vi "FestoCPX.DO.Data.Fglb.vi"(6 "Config":T1[](array[typedef]), 7 "state (get all)":T4=enum."get", 8 "error in (no error)":errorcluster, 9 "State":bool[](array[boolean]), 10 "Outputs":T3[](array[typedef])) -> (0 "error out":errorcluster, 1 "changed?":bool, 2 "State out":bool[](array[boolean]))   [LabVIEW 2016]
uses:
  FestoCPX.DO.Data.Fglb.Action.ctl
  FestoCPX.DO.Signal.ctl
  FestoCPX.DO.Sets.ctl
  FestoCPX.DO.ctl
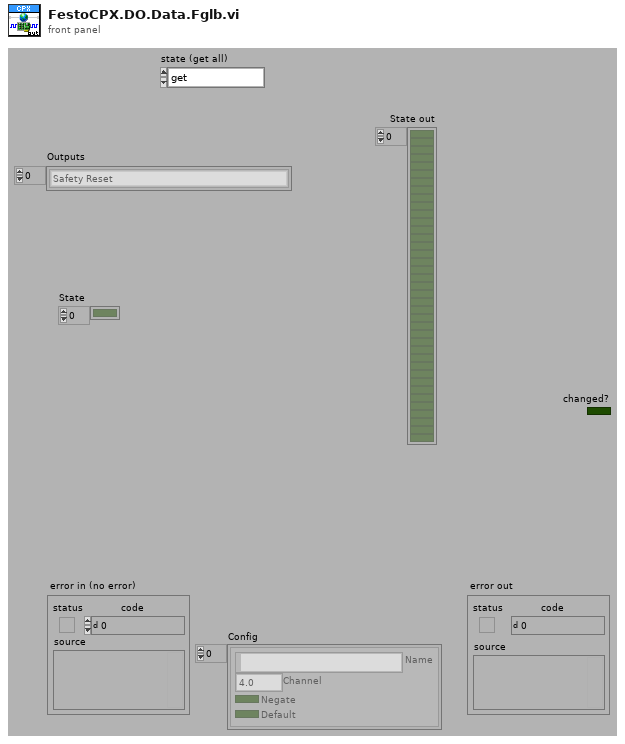
[diagram p1: front panel]
types:
  T1 = typedef "FestoCPX.DO.Sets.ctl" = cluster{"Name":string, "Channel":T2, "Negate":bool, "Default":bool}
  T2 = typedef "FestoCPX.DO.ctl" = enum16{"4.0", "4.1", "4.2", "4.3", "4.4", "4.5", "4.6", "4.7", "5.0", "5.1", "5.2", "5.3", "5.4", "5.5", "5.6", "5.7", "6.0", "6.1", "6.2", "6.3", "6.4", "6.5", "6.6", "6.7", "Q1K1", "Q1K2", "Q2K1", "Q2K2", "Q3K1", "Q3K2", "Q4K1", "Q4K2", "Q5K1", "Q5K2", "Q6K1", "Q6K2"}
  T3 = typedef "FestoCPX.DO.Signal.ctl" = enum16{"Safety Reset", "Air Main Valve", "Door Lock", "Button LED Start", "Button LED Stop", "Button LED Control", "Traffic LED Red", "Traffic LED Orange", "Traffic LED Green", "Horn", "Laser Interlock", "Laser Trigger", "Laser Fume Extractor", "Product Suction Gripper Slot 1 A", "Product Suction Gripper Slot 1 B", "Product Suction Gripper Slot 2 A", "Product Suction Gripper Slot 2 B", "Product Suction Gripper Slot 3 A", "Product Suction Gripper Slot 3 B", "Product Suction Gripper Slot 4 A", "Product Suction Gripper Slot 4 B", "Product Suction Gripper Final A", "Product Suction Gripper Final B", "Lamp", "Q1 Product Move Work", "Q1 Product Move Home", "Q2 Table Turn Work", "Q2 Table Turn Home", "Q3 Product Lift A", "Q3 Product Lift B", "Q4 Product Arm OK", "Q4 Product Arm NOK", "Q5 Product Arm Work", "Q6 Product BlowOut A", "Q6 Product BlowOut B"}
  T4 = typedef "FestoCPX.DO.Data.Fglb.Action.ctl" = enum16{"init", "set", "get", "check", "select", "reset"}
  T5 = cluster{"out":bool[], "Config":T1[], "changed":bool}
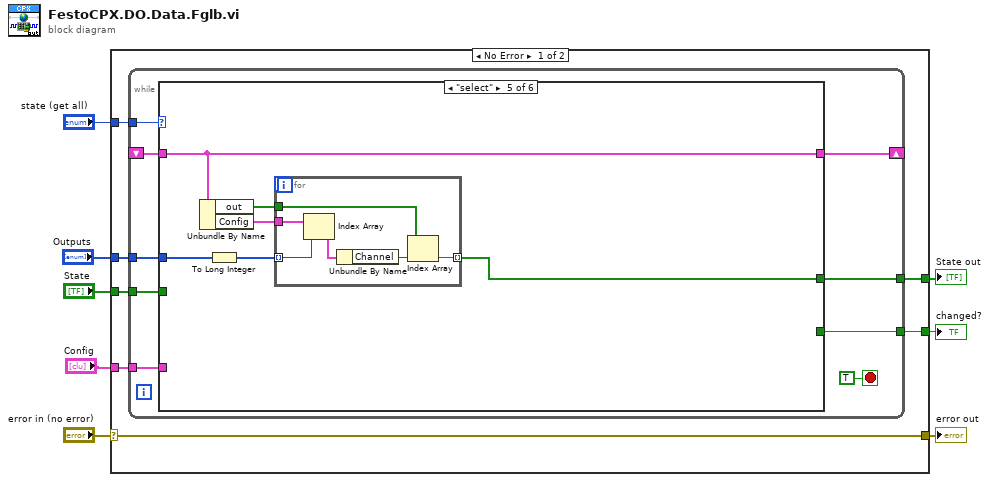
[diagram p0: block diagram]
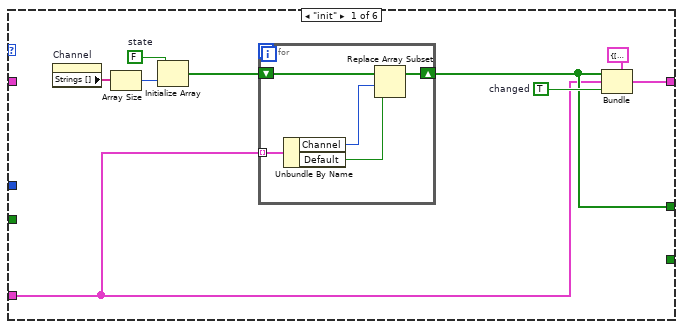
[diagram p2: hidden frame]
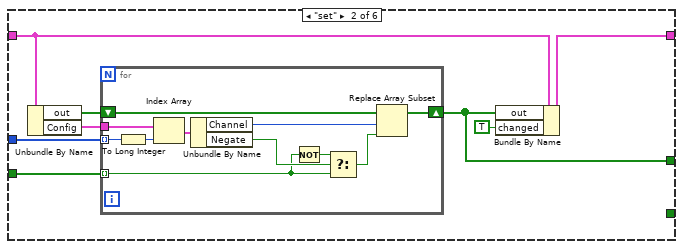
[diagram p3: hidden frame]
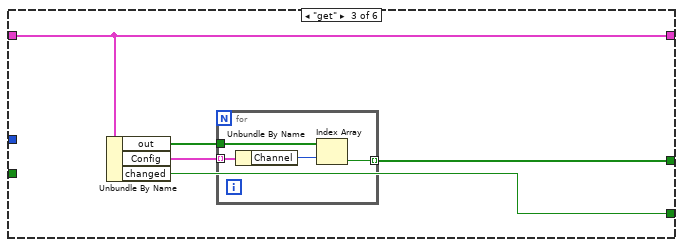
[diagram p4: hidden frame]
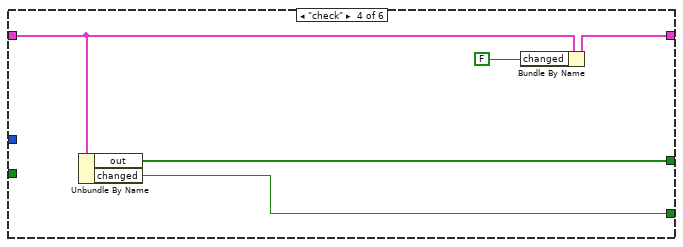
[diagram p5: hidden frame]
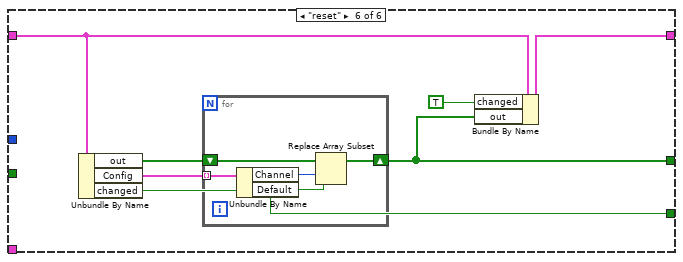
[diagram p6: hidden frame]
diagram:
  n1 = case shown="No Error" "error in (no error)" {
    selector: "error in (no error)" -> [w12 w94]
    tunnel: [w12 w94] -> w8
    tunnel: "state (get all)" -> [w15 _]
    tunnel: "Outputs" -> [w14 _]
    tunnel: "State" -> [w13 _]
    tunnel: "Config" -> [w11 _]
    tunnel: [w10 _] -> w3
    tunnel: [w9 _] -> w2
    frame No Error {
      n2 = while {
        tunnel: w15 -> [w23]
        shift-right: [w22] -> _
        shift-left: _ -> [w21]
        tunnel: w14 -> [w20]
        tunnel: w13 -> [w19]
        tunnel: w11 -> [w18]
        tunnel: [w17] -> w10
        tunnel: [w16] -> w9
        stop <- TRUE stop-if-true
        n3 = case shown="\"select\"" w23 {
          tunnel: [w32 w40 w62 w69 w75 w88] -> w22
          tunnel: w21 -> [_ w41 w62 w70 w75 w89]
          tunnel: w20 -> [_ w46 _ _ w72 _]
          tunnel: w19 -> [_ w45 _ _ _ _]
          tunnel: w18 -> [w25 _ _ _ _ _]
          tunnel: [w26 w39 w58 w71 w76 w85] -> w17
          tunnel: [_ _ w61 w67 _ w86] -> w16
          frame "init" {
            w28 = FALSE  # state
            w33 = TRUE  # changed
            n4 = property on="Channel" class="Enum (strict)"() -> ("Strings []"=w30:string[])  [unwired: 2 in, 2 out]
            n5 = Array Size(array=w30) -> (size(s)=w29:i32)
            n6 = Initialize Array(w28, w29) -> (w27:bool[])
            n7 = for {
              shift-right: [w37] -> w26
              shift-left: w27 -> [w38]
              tunnel: w25 -> [w34] mode=indexing
              n8 = Unbundle By Name(w34) -> ("Channel"=w35:T2, "Default"=w36:bool)
              n9 = Replace Array Subset(array=w38, new element=w36, index=w35) -> (w37:bool[])
            }
            n10 = Bundle(cluster=T5 {"out"=[], "Config"=[], "changed"=FALSE}, "out"=w26, "Config"=w25, "changed"=w33) -> (w32:T5)
          }
          frame "set" {
            n11 = Unbundle By Name(w41) -> ("out"=w43:bool[], "Config"=w44:T1[])
            n12 = for {
              tunnel: w44 -> [w55]
              shift-right: [w57] -> w39
              shift-left: w43 -> [w51]
              tunnel: w46 -> [w47] mode=indexing
              tunnel: w45 -> [w52] mode=indexing
              n13 = To Long Integer(number=w47) -> (32bit integer=w48:i32)
              n14 = Index Array(array=w55, index=w48) -> (element=w54:T1)
              n15 = Unbundle By Name(w54) -> ("Channel"=w50:T2, "Negate"=w53:bool)
              n16 = Not(x=w52) -> (.not. x?=w56:bool)
              n17 = Select(t=w56, s=w53, f=w52) -> (s? t:f=w49:bool)
              n18 = Replace Array Subset(array=w51, new element=w49, index=w50) -> (w57:bool[])
            }
            n19 = Bundle By Name(cluster=w41, "out"=w39, "changed"=TRUE) -> (w40:T5)
          }
          frame "get" {
            n20 = Unbundle By Name(w62) -> ("out"=w60:bool[], "Config"=w59:T1[], "changed"=w61:bool)
            n21 = for {
              tunnel: w60 -> [w66]
              tunnel: w59 -> [w65] mode=indexing
              tunnel: [w63] -> w58 mode=indexing
              n22 = Unbundle By Name(w65) -> ("Channel"=w64:T2)
              n23 = Index Array(array=w66, index=w64) -> (element=w63:bool)
            }
          }
          frame "check" {
            n24 = Unbundle By Name(w70) -> ("out"=w71:bool[], "changed"=w67:bool)
            n25 = Bundle By Name(cluster=w70, "changed"=FALSE) -> (w69:T5)
          }
          frame "select" {
            n26 = Unbundle By Name(w75) -> ("out"=w77:bool[], "Config"=w74:T1[])
            n27 = To Long Integer(number=w72) -> (32bit integer=w73:i32[])
            n28 = for {
              tunnel: w73 -> [w80] mode=indexing
              tunnel: w77 -> [w83]
              tunnel: [w82] -> w76 mode=indexing
              tunnel: w74 -> [w81]
              n29 = Index Array(array=w81, index=w80) -> (element=w79:T1)
              n30 = Unbundle By Name(w79) -> ("Channel"=w78:T2)
              n31 = Index Array(array=w83, index=w78) -> (element=w82:bool)
            }
          }
          frame "reset" {
            n32 = Unbundle By Name(w89) -> ("out"=w85:bool[], "Config"=w84:T1[], "changed"=w86:bool)
            n33 = for {
              shift-right: [w93] -> _
              shift-left: w85 -> [w93]
              tunnel: w84 -> [w92] mode=indexing
              n34 = Unbundle By Name(w92) -> ("Channel"=w91:T2, "Default"=w90:bool)
              n35 = Replace Array Subset(array=w93, new element=w90, index=w91) -> ()  [unwired: 1 out]
            }
            n36 = Bundle By Name(cluster=w89, "changed"=TRUE, "out"=w85) -> (w88:T5)
          }
        }
      }
    }
    frame Error {
    }
  }
  "error out" <- w8
  "State out" <- w3
  "changed?" <- w2
